vi "SetResetScreen.vi"(8 "error in (no error)":errorcluster, 11 "VISA resource name":refnum<visa-resource-name>) -> (0 "error out":errorcluster, 2 "8800 response":string, 3 "VISA resource name out":refnum<visa-resource-name>)   [LabVIEW 2023, in "Thermotron 8800.lvlib"]
doc: "SCRR\nCommand name: Reset screen\nCommand type: Control\nDescription: Forces the 8800 to go to the main screen.\nSyntax: SCRR\nData type: No data\nOperation example: SCRR\n8800 response: Switches the 8800’s current screen to the main screen."
uses:
  Thermotron 8800.lvlib
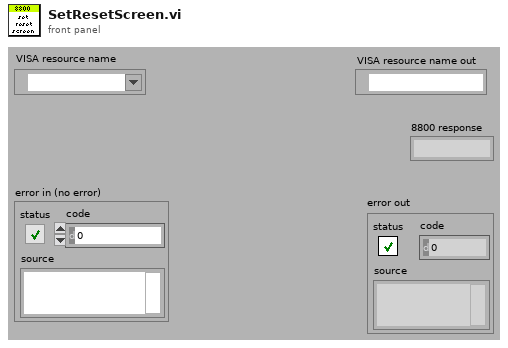
[diagram p1: front panel]
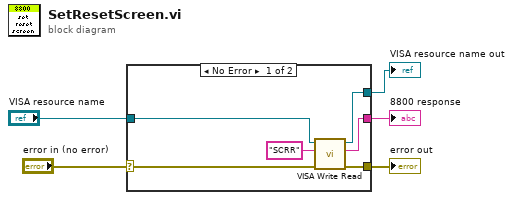
[diagram p0: block diagram]
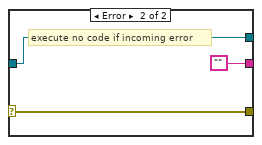
[diagram p2: hidden frame]
diagram:
  n1 = case shown="No Error" "error in (no error)" {
    selector: "error in (no error)" -> [w7 w14]
    tunnel: "VISA resource name" -> [w11 w13]
    tunnel: [w10 w13] -> w3
    tunnel: [w9 w14] -> w4
    tunnel: [w8 "" ("read buffer")] -> w2
    frame No Error {
      n2 = call "VISA Write Read.vi"("error in (no error)"=w7, "8800 Command"="SCRR", "VISA Refnum in"=w11) -> ("error out"=w9:errorcluster, "read buffer"=w8:string, "VISA Refnum out"=w10:refnum<visa-resource-name>)  [unwired: 6 in]
    }
    frame Error {
      # "execute no code if incoming error"
    }
  }
  "VISA resource name out" <- w3
  "error out" <- w4
  "8800 response" <- w2
